vi "Write Limit Volt.vi"(8 "error in":errorcluster, 10 "OverVoltage_Protect":dbl, 11 "57XX in":refnum<class "57XX.lvclass">) -> (0 "error out":errorcluster, 3 "57XX out":refnum<class "57XX.lvclass">)   [LabVIEW 2019, in "57XX.lvlib" / "57XX.lvclass"]
uses:
  Library/57XX.lvclass
  C:/Users/Public/Documents/Development/builds/Instruments/PowerSupply.lvlibp/Library/PowerSupply.lvclass
  builds/Instruments/PowerSupply.lvlibp/Library/PowerSupply.lvclass
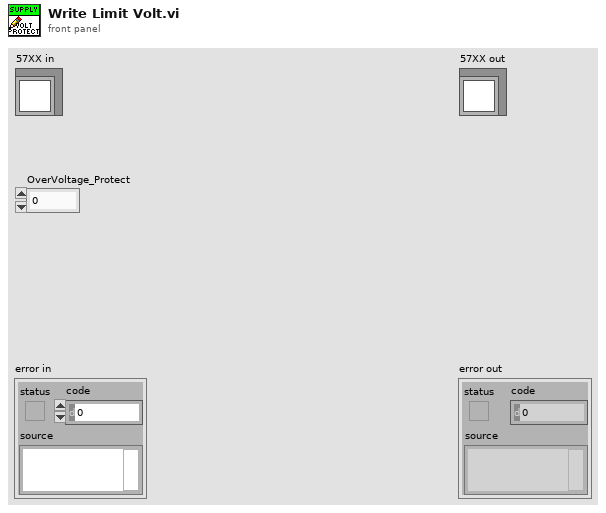
[diagram p1: front panel]
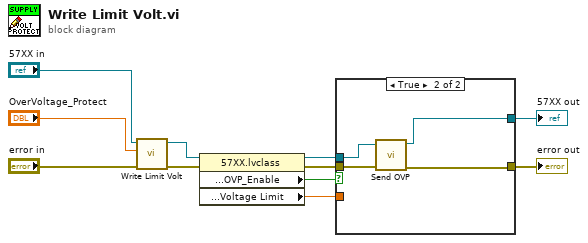
[diagram p0: block diagram]
diagram:
  n1 = call-parent "Write Limit Volt.vi"("error in"="error in", "OverVoltage_Protect"="OverVoltage_Protect", "PowerSupply in"="57XX in") -> ("error out"=w7:errorcluster, "PowerSupply out"=w8:refnum<class "57XX.lvclass">)  [unwired: 7 in]
  n2 = property class="57XX.lvclass"(reference=w8, error in=w7) -> (reference out=w5:refnum<class "57XX.lvclass">, error out=w3:errorcluster, "Accessors:Setting:Protection:OVP_Enable"=w6:bool, "Accessors:Setting:Protection:Voltage Limit"=w1:dbl)
  n3 = case shown="True" w6 {
    tunnel: w5 -> [w13 w16]
    tunnel: [w13 w14] -> w4
    tunnel: w3 -> [w12 w17]
    tunnel: [w12 w15] -> w2
    tunnel: w1 -> [_ _]
    frame False {
    }
    frame True {
      n4 = call "Send OVP.vi"("error in (no error)"=w17, "57XX in"=w16) -> ("error out"=w15:errorcluster, "57XX out"=w14:refnum<class "57XX.lvclass">)  [unwired: 8 in]
    }
  }
  "error out" <- w2
  "57XX out" <- w4
